vi "UsrProfiles-Obtain default profile.vi"(11 "Config Files Folder Path":path) -> (3 "\"Default user\" or \"Previous session\" profile's filepath":path)   [LabVIEW 2020]
uses:
  Global Variables/General Globals.vi
panel:
  out "\"Default user\" or \"Previous session\" profile's file name":string
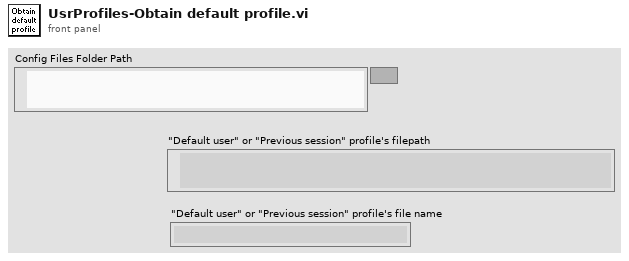
[diagram p1: front panel]
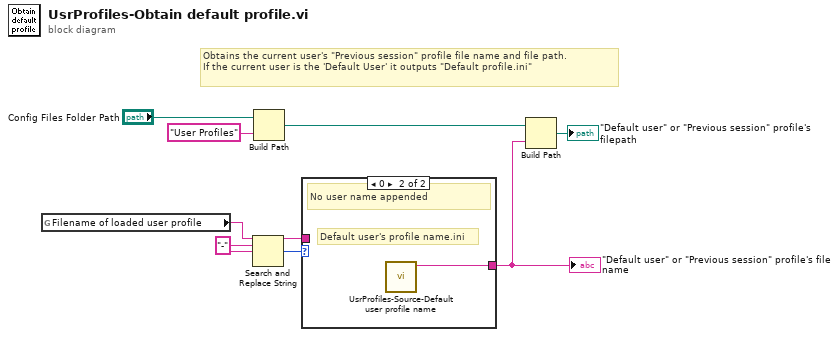
[diagram p0: block diagram]
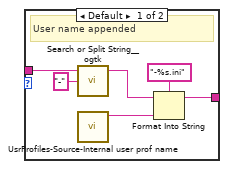
[diagram p2: hidden frame]
diagram:
  w4 = "-" ("search string")
  # "Obtains the current user's \"Previous session\" profile file name and file path.\nIf the current user is the 'Default User' it outputs \"Default profile.ini\""
  n1 = global read "General Globals.vi" "Filename of loaded user profile"() -> (w5:string)
  n2 = Search and Replace String(input string=w5, search string=w4, replace string=w4) -> (result string=w2:string, number of replacements=w3:i32)  [unwired: 5 in, 2 out]
  n3 = Build Path(base path="Config Files Folder Path", name or relative path="User Profiles") -> (appended path=w8:path)
  n4 = case shown="0" w3 {
    tunnel: w2 -> [w14 _]
    tunnel: [w10 w16] -> w1
    frame Default {
      # "User name appended"
      n5 = call <userlib>:"Search or Split String__ogtk.vi"("search string/char (-)"="-", "string"=w14) -> ("substring before match"=w13:string)  [unwired: 1 in, 2 out]
      n6 = call "UsrProfiles-Source-Internal user prof name.vi"() -> ("Previous session profile name"=w11:string)  [unwired: 11 in]
      n7 = Format Into String(format string="-%s.ini", initial string=w13, w11) -> (resulting string=w10:string)  [unwired: 1 in, 1 out]
    }
    frame 0 {
      # "Default user's profile name.ini"
      # "No user name appended"
      n8 = call "UsrProfiles-Source-Default user profile name.vi"() -> ("Default user's profile file name & extension"=w16:string)  [unwired: 11 in]
    }
  }
  "\"Default user\" or \"Previous session\" profile's file name" <- w1
  n9 = Build Path(base path=w8, name or relative path=w1) -> (appended path=→"\"Default user\" or \"Previous session\" profile's filepath":path)
